vi "test.vi"   [LabVIEW 2012]
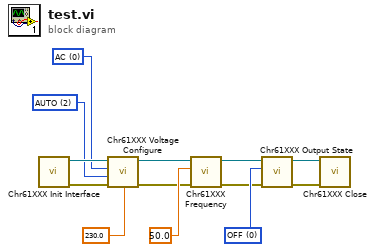
[diagram p0: block diagram]
diagram:
  w5 = 2 items=["LOW", "HIGH", "AUTO"] ("voltage range")
  w6 = 0 items=["AC", "DC"] ("voltage type")
  w9 = u16 0 items=["OFF", "ON"] ("state")
  n1 = call <instrlib>:"Chr61XXX Init Interface.vi"() -> ("error out"=w4:errorcluster, "instrument handle out"=w10:refnum<k15>)  [unwired: 9 in, 1 out]
  n2 = call <instrlib>:"Chr61XXX Voltage Configure.vi"("voltage"=230.0, "error in (no error)"=w4, "voltage range"=w5, "voltage type"=w6, "instrument handle"=w10) -> ("error out"=w3:errorcluster, "instrument handle out"=w11:refnum<k15>)  [unwired: 5 in]
  n3 = call <instrlib>:"Chr61XXX Frequency.vi"("error in (no error)"=w3, "frequency"=50.0, "instrument handle"=w11) -> ("error out"=w2:errorcluster, "instrument handle out"=w8:refnum<k15>)  [unwired: 7 in]
  n4 = call <instrlib>:"Chr61XXX Output State.vi"("error in (no error)"=w2, "state"=w9, "instrument handle"=w8) -> ("error out"=w1:errorcluster, "instrument handle out"=w7:refnum<k15>)  [unwired: 7 in]
  n5 = call <instrlib>:"Chr61XXX Close.vi"("error in (no error)"=w1, "instrument handle"=w7) -> ()  [unwired: 9 in, 1 out]
